vi "Read Channel Refnum.vi"(8 "error in (no error)":errorcluster, 11 "Channel":T1) -> (0 "error out":errorcluster, 2 "LIBSSH2_CHANNEL*":u64)   [LabVIEW 2013, in "libssh2.lvlib"]
uses:
  libssh2.lvlib
  Channel Refnum.ctl
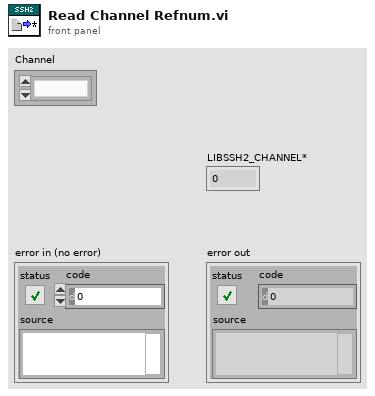
[diagram p1: front panel]
types:
  T1 = typedef "libssh2.lvlib/Channel Refnum.ctl" = refnum<k1>
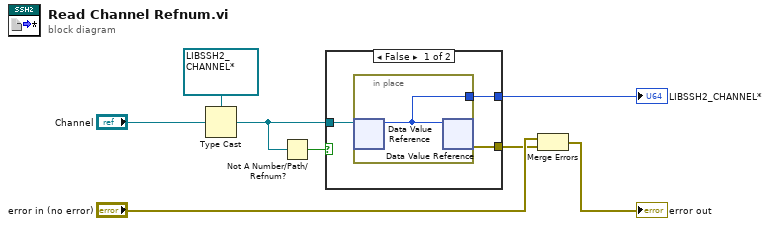
[diagram p0: block diagram]
diagram:
  n1 = Type Cast(type=refnum<data-value> refnum ("data value reference"), x="Channel") -> (*(type *) &x=w2:refnum<data-value>)
  n2 = Not A Number/Path/Refnum?(number/path/refnum=w2) -> (NaN/Path/Refnum?=w1:bool)
  n3 = case shown="False" w1 {
    tunnel: w2 -> [w11 _]
    tunnel: [w10 _] -> w7
    tunnel: [w9 _] -> w3
    frame False {
      n4 = in-place {
        in-place-border: [w12] -> w10
        n5 = in-place-dvr #1(w11) -> (w12:u64)  [unwired: 1 out]
        n6 = in-place-dvr #1(w12) -> (w9:errorcluster)  [unwired: 1 out]
      }
    }
    frame True {
    }
  }
  "LIBSSH2_CHANNEL*" <- w7
  n7 = Merge Errors("error in (no error)", w3) -> (→"error out":errorcluster)
